vi "setAvalibleHardwareList.vi"(8 "error in (no error)":errorcluster, 11 "HWController in":refnum<class "HWController.lvclass">) -> (0 "error out":errorcluster, 3 "HWController out":refnum<class "HWController.lvclass">)   [LabVIEW 2009, in "Hardware.lvlib" / "HWControllers.lvlib" / "HWController.lvclass"]
doc: "Sets the Available HW list.\n\nThis hardware can be used for an experiment"
uses:
  HWController.lvclass
  HWController.lvclass/HWController.ctl
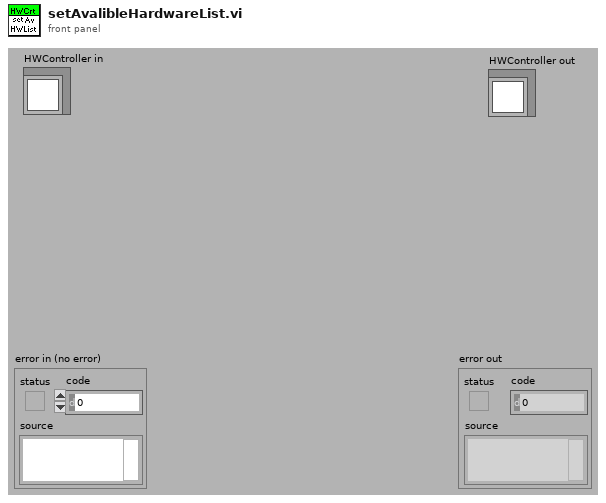
[diagram p1: front panel]
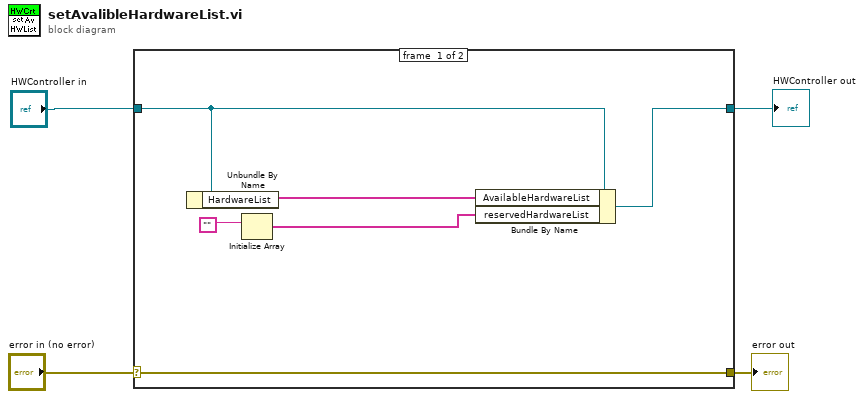
[diagram p0: block diagram]
diagram:
  n1 = case shown="No Error" "error in (no error)" {
    selector: "error in (no error)" -> [w10 w12]
    tunnel: [w10 w12] -> w3
    tunnel: [w7 w11] -> w1
    tunnel: "HWController in" -> [w8 w11]
    frame #0 {
      n2 = Unbundle By Name(w8) -> ("HardwareList"=w9:string[])
      n3 = Initialize Array("") -> (w6:string[])  [unwired: 1 in]
      n4 = Bundle By Name(cluster=w8, "AvailableHardwareList"=w9, "reservedHardwareList"=w6) -> (w7:refnum<class "HWController.lvclass">)
    }
    frame #1 {
    }
  }
  "error out" <- w3
  "HWController out" <- w1
